vi "Accels to Roll_Pitch.vi"(2 "az":sgl=1.0, 3 "ay":sgl, 4 "ax":sgl) -> (0 "Pitch (deg)":sgl, 1 "Roll (deg)":sgl)   [LabVIEW 2017]
panel:
  # "PN 23/03/18"
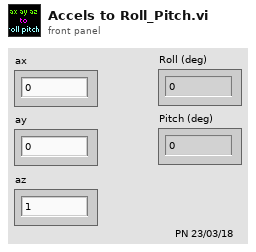
[diagram p1: front panel]
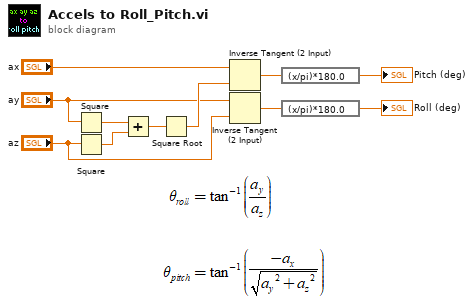
[diagram p0: block diagram]
diagram:
  n1 = Square(x="ay") -> (x^2=w10:sgl)
  n2 = Square(x="az") -> (x^2=w11:sgl)
  n3 = Add(x=w10, y=w11) -> (x+y=w9:sgl)
  n4 = Square Root(x=w9) -> (sqrt(x)=w4:sgl)
  n5 = Inverse Tangent (2 Input)(1:w4, 2:"ax") -> (0:w8:sgl)
  n6 = Inverse Tangent (2 Input)(1:"az", 2:"ay") -> (0:w7:sgl)
  n7 = expression code="(x/pi)*180.0" ("radians to degrees")(w8) -> (→"Pitch (deg)":sgl)
  n8 = expression code="(x/pi)*180.0" ("radians to degrees")(w7) -> (→"Roll (deg)":sgl)
